vi "Enable Input.vi"(7 "Enable Input (F: Disable)":bool, 8 "error in (no error)":errorcluster, 9 "Operation Type (0: Set)":i32(ring) items=["Set", "Get"], 10 "Channel (1: Channel 1)":i32(ring)=1 items=["Channel 1"=1, "Channel 2"=2], 11 "VISA resource name":refnum<visa-resource-name>) -> (0 "error out":errorcluster, 2 "Input Enabled?":bool, 3 "VISA resource name out":refnum<visa-resource-name>)   [LabVIEW 2017, in "Keysight B2980 Series.lvlib"]
doc: "Enables or disables the current or charge input.\n\n<b>Note(s):</b>\nFor models B2981A and B2983A, only current measurement is supported."
uses:
  Keysight B2980 Series.lvlib
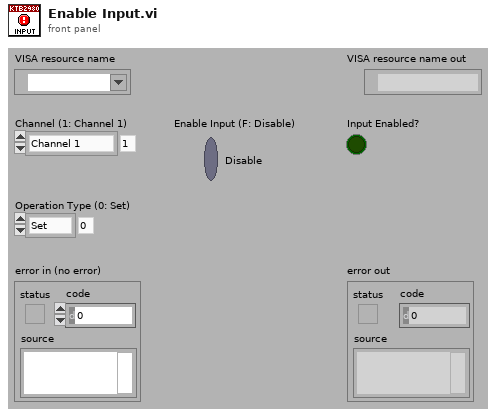
[diagram p1: front panel]
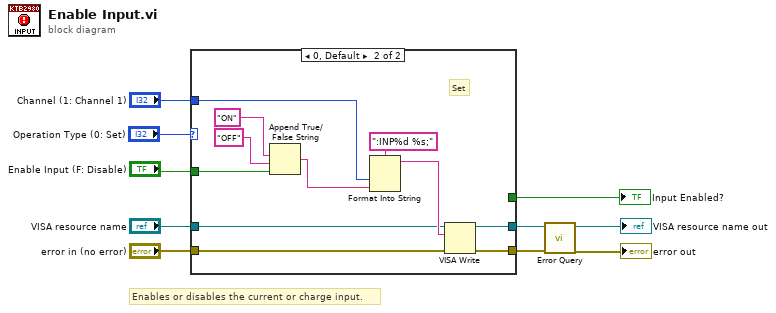
[diagram p0: block diagram]
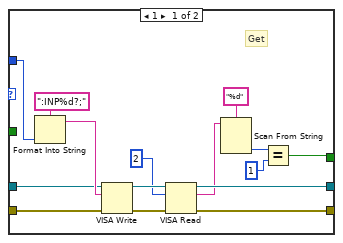
[diagram p2: hidden frame]
diagram:
  # "Enables or disables the current or charge input."
  n1 = case shown="0, Default" "Operation Type (0: Set)" {
    tunnel: "Enable Input (F: Disable)" -> [_ w34]
    tunnel: "Channel (1: Channel 1)" -> [w11 w32]
    tunnel: "VISA resource name" -> [w23 w29]
    tunnel: "error in (no error)" -> [w22 w28]
    tunnel: [w18 w27] -> w6
    tunnel: [w17 w26] -> w5
    tunnel: [w12 _] -> w1
    frame 1 {
      # "Get"
      n2 = Format Into String(format string=":INP%d?;", w11) -> (resulting string=w24:string)  [unwired: 2 in, 1 out]
      n3 = VISA Write(VISA resource name=w23, write buffer=w24, error in (no error)=w22) -> (VISA resource name out=w21:refnum<visa-resource-name>, error out=w20:errorcluster)  [unwired: 1 out]
      n4 = VISA Read(VISA resource name=w21, byte count=u32 2, error in (no error)=w20) -> (VISA resource name out=w18:refnum<visa-resource-name>, read buffer=w16:string, error out=w17:errorcluster)  [unwired: 1 out]
      n5 = Scan From String(format string="%d", input string=w16) -> (output 1=w14:i32)  [unwired: 2 in, 4 out]
      n6 = Equal?(x=w14, y=1) -> (x = y?=w12:bool)
    }
    frame 0, Default {
      # "Set"
      n7 = Append True/False String(1:w34, 2:"OFF", 3:"ON") -> (0:w31:string)  [unwired: 1 out]
      n8 = Format Into String(format string=":INP%d %s;", w32, w31) -> (resulting string=w30:string)  [unwired: 2 in, 1 out]
      n9 = VISA Write(VISA resource name=w29, write buffer=w30, error in (no error)=w28) -> (VISA resource name out=w27:refnum<visa-resource-name>, error out=w26:errorcluster)  [unwired: 1 out]
    }
  }
  "Input Enabled?" <- w1
  n10 = call "Error Query.vi"("error in (no error)"=w5, "VISA resource name"=w6) -> ("error out"=→"error out":errorcluster, "VISA resource name out"=→"VISA resource name out":refnum<visa-resource-name>)  [unwired: 8 out]
